vi "Read Spec Page Path.vi"(8 "error in (no error)":errorcluster, 11 "NIVS_CDW_MetaDataObj in":refnum<class "NIVS_ScriptedModuleTemplate_MetaDataObj.lvclass">) -> (0 "error out":errorcluster, 2 "Path to Spec Page VI":path, 3 "NIVS_CDW_MetaDataObj out":refnum<class "NIVS_ScriptedModuleTemplate_MetaDataObj.lvclass">)   [LabVIEW 2015, in "NIVS_ScriptedModuleTemplate_MetaDataObj.lvclass"]
uses:
  NIVS_ScriptedModuleTemplate_MetaDataObj.lvclass
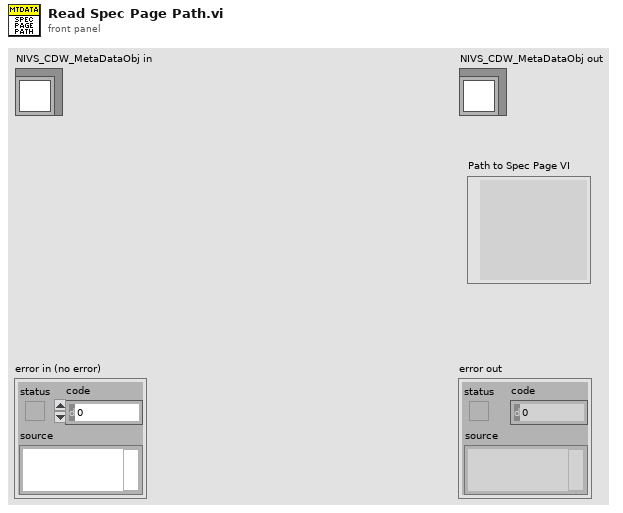
[diagram p1: front panel]
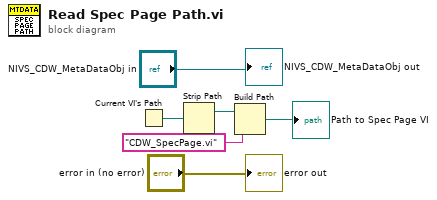
[diagram p0: block diagram]
diagram:
  n1 = Current VI's Path() -> (path=w4:path)
  n2 = Strip Path(path=w4) -> (stripped path=w3:path)  [unwired: 1 out]
  n3 = Build Path(base path=w3, name or relative path="CDW_SpecPage.vi") -> (appended path=→"Path to Spec Page VI":path)
  "error out" <- "error in (no error)"
  "NIVS_CDW_MetaDataObj out" <- "NIVS_CDW_MetaDataObj in"
